vi "Get Exported Routines.vi"(8 "error in (no error)":errorcluster, 11 "Item Ref in":T5 format="%.0x") -> (0 "error out":errorcluster, 2 "Routines":T1 {"Routine Array"."Stop Parameters"."Response"."Byte Order" items=["Little Endian", "Big Endian"]; "Routine Array"."Stop Parameters"."Response"."Data Type" items=["Signed", "Unsigned", "IEEE Float"]; "Routine Array"."Stop Parameters"."Cmd"."Byte Order" items=["Little Endian", "Big Endian"]; "Routine Array"."Stop Parameters"."Cmd"."Data Type" items=["Signed", "Unsigned", "IEEE Float"]; "Routine Array"."Request Parameters"."Response"."Byte Order" items=["Little Endian", "Big Endian"]; "Routine Array"."Request Parameters"."Response"."Data Type" items=["Signed", "Unsigned", "IEEE Float"]; "Routine Array"."Request Parameters"."Cmd"."Byte Order" items=["Little Endian", "Big Endian"]; "Routine Array"."Request Parameters"."Cmd"."Data Type" items=["Signed", "Unsigned", "IEEE Float"]; "Routine Array"."Start Parameters"."Response"."Byte Order" items=["Little Endian", "Big Endian"]; "Routine Array"."Start Parameters"."Response"."Data Type" items=["Signed", "Unsigned", "IEEE Float"]; "Routine Array"."Start Parameters"."Cmd"."Byte Order" items=["Little Endian", "Big Endian"]; "Routine Array"."Start Parameters"."Cmd"."Data Type" items=["Signed", "Unsigned", "IEEE Float"]}, 3 "Section Ref out":T5 format="%.0x")   [LabVIEW 2015, in "Diagnostics Addon System Explorer.lvlib"]
uses:
  Diagnostics Addon System Explorer.lvlib
  <vilib>/NI Veristand/Custom Device API/Custom Device Item Ref.ctl
  Shared/Types/Exported Routines Cluster.ctl
  Shared/Types/Routine Paramaters.ctl
  Shared/Types/Command Response Signals.ctl
  Shared/Types/Signal Parameters.ctl
  ID FG.vi
  Export CmdResp Pair.vi
  Get Signals.vi
  Type FG.vi
  Signal Parameters FG.vi
  <vilib>/NI Veristand/Custom Device API/NI VeriStand - Get Item Property.vi
  <vilib>/NI Veristand/Custom Device API/Get Item Property (U32).vi
  <vilib>/NI Veristand/Custom Device API/NI VeriStand - Set Item Property.vi
  <vilib>/NI Veristand/Custom Device API/Set Item Property (U32).vi
  Shared/SubVIs/GUID Lookup.vi
  <vilib>/NI Veristand/Custom Device API/NI VeriStand - Get Custom Device Channel Data.vi
  <vilib>/NI Veristand/Custom Device API/Get Item Property (String).vi
  <vilib>/NI Veristand/Custom Device API/Get Item Property (Double).vi
  <vilib>/NI Veristand/Custom Device API/Set Item Property (String).vi
  <vilib>/NI Veristand/Custom Device API/Set Item Property (Double).vi
  <vilib>/NI Veristand/Custom Device Tools/Custom Device Utility Library/NI VeriStand - Search for Item by GUID.vi
  <vilib>/NI Veristand/Custom Device API/NI VeriStand - Get Item Data.vi
  <vilib>/NI Veristand/Custom Device Tools/Custom Device Utility Library/Custom Device Utility Library.lvlib
  <vilib>/NI Veristand/Custom Device API/Custom Device API.lvlib
  Shared/Diagnostics Addon Shared.lvlib
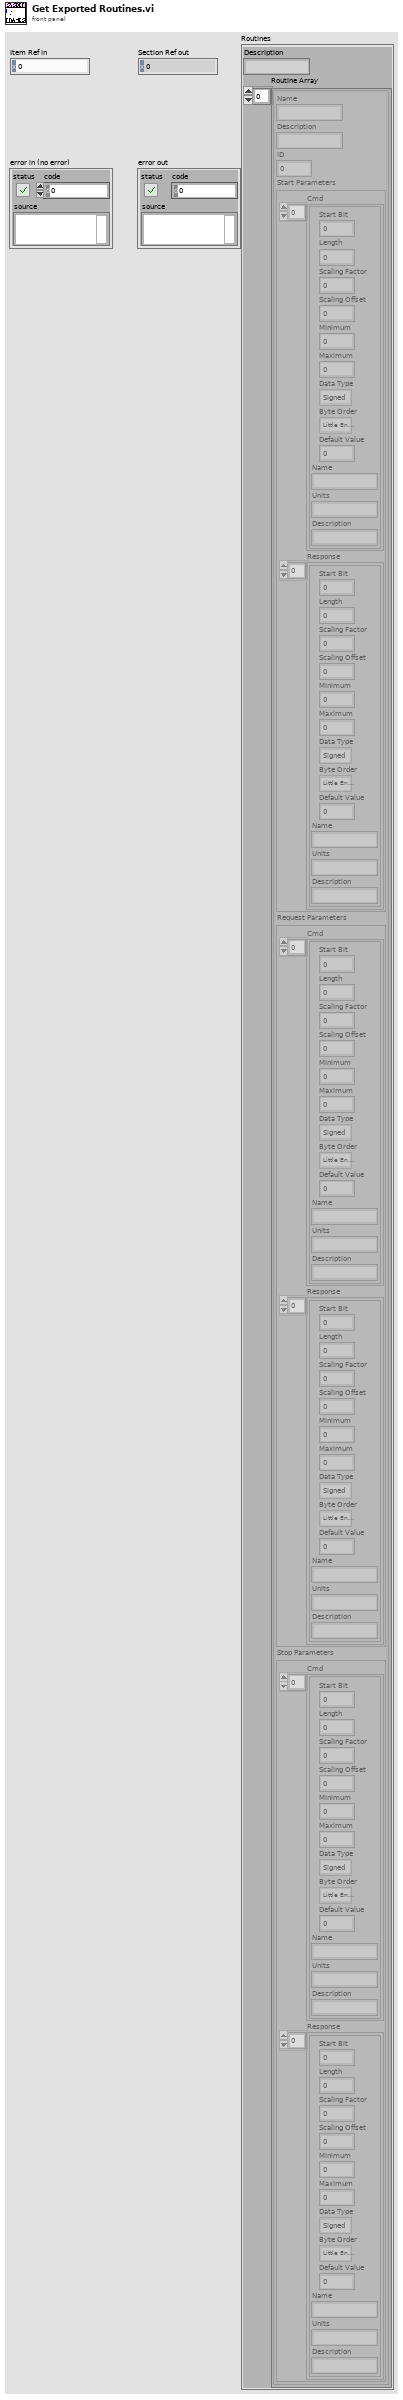
[diagram p1: front panel]
types:
  T1 = typedef "Diagnostics Addon Shared.lvlib/Exported Routines Cluster.ctl" = cluster{"Description":string, "Routine Array":T2[]}
  T2 = typedef "Diagnostics Addon Shared.lvlib/Routine Paramaters.ctl" = cluster{"Name":string, "Description":string, "ID":u16, "Start Parameters":T3, "Request Parameters":T3, "Stop Parameters":T3}
  T3 = typedef "Diagnostics Addon Shared.lvlib/Command Response Signals.ctl" = cluster{"Cmd":T4[], "Response":T4[]}
  T4 = typedef "Diagnostics Addon Shared.lvlib/Signal Parameters.ctl" = cluster{"Start Bit":u8, "Length":u8, "Scaling Factor":dbl, "Scaling Offset":dbl, "Minimum":dbl, "Maximum":dbl, "Data Type":u32, "Byte Order":u32, "Default Value":dbl, "Name":string, "Units":string, "Description":string}
  T5 = typedef "Custom Device API.lvlib/Custom Device Item Ref.ctl" = u64
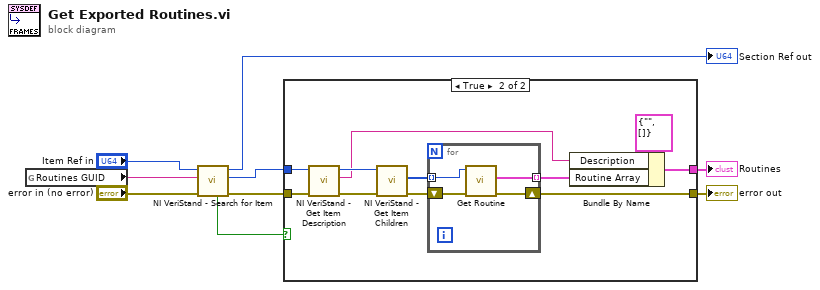
[diagram p0: block diagram]
diagram:
  n1 = global read "GUID Lookup.vi" "Routines GUID"() -> (w2:string)
  n2 = call-poly <vilib>:"NI VeriStand - Search for Item.vi"("error in"="error in (no error)", "Item GUID"=w2, "Section Ref in"="Item Ref in") -> ("error out"=w5:errorcluster, "Item Ref"=w4:T5, "Section Ref out"=→"Section Ref out":T5, "Found"=w3:bool)  [unwired: 5 in]
  n3 = case shown="True" w3 {
    tunnel: [_ w13] -> w1
    tunnel: [w10 w21] -> w6
    tunnel: w5 -> [w10 w16]
    tunnel: w4 -> [_ w18]
    frame False {
    }
    frame True {
      n4 = call <vilib>:"NI VeriStand - Get Item Description.vi"("error in (no error)"=w16, "Item Ref in"=w18) -> ("error out"=w15:errorcluster, "Description"=w14:string, "Item Ref out"=w17:T5)  [unwired: 7 out]
      n5 = call <vilib>:"NI VeriStand - Get Item Children.vi"("error in (no error)"=w15, "Item Ref in"=w17) -> ("error out"=w20:errorcluster, "Child Refs"=w19:T5[])  [unwired: 6 in, 2 out]
      n6 = for {
        tunnel: w19 -> [w25] mode=indexing
        shift-right: [w23] -> w21
        shift-left: w20 -> [w24]
        tunnel: [w22] -> w12 mode=indexing
        n7 = call "Get Routine.vi"("error in (no error)"=w24, "Item Ref in"=w25) -> ("error out"=w23:errorcluster, "Routine"=w22:T2)  [unwired: 7 in, 1 out]
      }
      n8 = Bundle By Name(cluster=T1 {"Description"="", "Routine Array"=[]} ("Routines"), "Description"=w14, "Routine Array"=w12) -> (w13:T1)
    }
  }
  "error out" <- w6
  "Routines" <- w1
